vi "chooseOffensivePlay.vi"(8 "error in (no error)":errorcluster, 11 "Game":refnum<class "Game.lvclass">) -> (0 "error out":errorcluster, 2 "passFinishConditions":bool[](array[boolean]), 3 "Game out":refnum<class "Game.lvclass">, 4 "passdebug":T2[](array[typedef]), 5 "debugOffensivePlayFinished":T1[](array[typedef]))   [LabVIEW 2020, in "Game.lvclass"]
uses:
  Game.lvclass
  Team_class/OffensivePlay.ctl
  5RobotsPassGamePlay_class/PassFinishBallVelConditionDegub.ctl
  5RobotsPassGamePlay_class/PassFinishReceiverDistanceToBallConditionDebug.ctl
  Referee_class/command_interpreted.ctl
  Game.lvclass/Game.ctl
  Team_class/Team.lvclass/Team.ctl
  Referee_class/Referee.lvclass/Referee.ctl
  StopOffensivePlay_class/StopOffensivePlay.lvclass
  PreparePenaltyEnemyPlay_class/PreparePenaltyEnemyPlay.lvclass
  EnemyPossessionAtEnemyFieldPlay_class/EnemyPossessionAtEnemyFieldPlay.lvclass
  EnemyPossessionAtOurFieldPlay_class/EnemyPossessionAtOurFieldPlay.lvclass
  PreparePenaltyAllyPlay_class/PreparePenaltyAllyPlay.lvclass
  KickPenaltyAllyPlay_class/KickPenaltyAllyPlay.lvclass
  PrepareKickoffAllyPlay_class/PrepareKickoffAllyPlay.lvclass
  PrepareKickoffEnemyPlay_class/PrepareKickoffEnemyPlay.lvclass
  SimplePass_class/SimplePass.lvclass
  PreparePassPlay_class/PreparePassPlay.lvclass
  PrepareRollToPassPlay_class/PrepareRollToPassPlay.lvclass
  PrepareDoublePassPlay_class/PrepareDoublePassPlay.lvclass
  PrepareTriplePassPlay_class/PrepareTriplePassPlay.lvclass
  PassToStriker_class/PassToStriker.lvclass
  PassTo2ndStriker_class/PassTo2ndStriker.lvclass
  KeeperPassToStrikerPlay_class/KeeperPassToStrikerPlay.lvclass
  TableWithStrikerPlay_class/TableWithStrikerPlay.lvclass
  TableWith2ndStrikerPlay_class/TableWith2ndStrikerPlay.lvclass
  ABCPassPlay_class/ABCPassPlay.lvclass
  ACBPassPlay_class/ACBPassPlay.lvclass
  DirectKickPlay_class/DirectKickPlay.lvclass
  DirectEnemyPlay_class/DirectEnemyPlay.lvclass
  NormalGamePlay_class/NormalGamePlay.lvclass
  PrepareKeeperPassPlay_class/PrepareKeeperPassPlay.lvclass
  PreparePassInGame1_class/PreparePassInGame1.lvclass
  5RobotsPassGamePlay_class/5RobotsPassGamePlay.lvclass
  5PreparePassGamePlay_class/5PreparePassGamePlay.lvclass
  5RobotsNormalGamePlay_class/5RobotsNormalGamePlay.lvclass
  5RobotsKeeperGame_class/5RobotsKeeperGame.lvclass
  TestPlay_class/TestPlay.lvclass
  BallOutOfFieldPlay_class/BallOutOfFieldPlay.lvclass
  Utilities_class/Utilities.lvclass
  Playbook_class/Playbook.lvclass/Playbook.ctl
  Playbook_class/Read offensive_plays.vi
  Playbook_class/Write offensive_plays.vi
  Read OffensiveTeam.vi
  Read Referee.vi
  Referee_class/Read command_interpreted.vi
  Team_class/Read OffensivePlay.vi
  Team_class/Write OffensivePlay.vi
  Write OffensiveTeam.vi
  Ally_class/Ally.lvclass
  Referee_class/Referee.lvclass
  Playbook_class/Playbook.lvclass
  Play_class/Play.lvclass
  IndirectEnemyPlay_class/IndirectEnemyPlay.lvclass
  PassPlay_class/PassPlay.lvclass
  HaltPlay_class/HaltPlay.lvclass
panel:
  in  "NewOffensivePlays":T3[](array[typedef])=[enum."TestPlay", enum."BallOutOfField", enum."StopOffensive", enum."Prepare Penalty Enemy", enum."PreparePenaltyAlly", enum."KickPenaltyAlly", enum."PrepareKickoffAlly", enum."PrepareKickoffEnemy", enum."DirectEnemy", enum."PreparePass", enum."EnemyPossesionAtOurField", enum."EnemyPossessionAtEnemyField", enum."5RobotsKeeperGame", enum."5RobotsPassGamePlay", enum."5PreparePassGame", enum."5RobotsNormalGamePlay"]
  in  "OldOffensivePlays":T3[](array[typedef])=[enum."TestPlay", enum."BallOutOfField", enum."StopOffensive", enum."Prepare Penalty Enemy", enum."PreparePenaltyAlly", enum."KickPenaltyAlly", enum."PrepareKickoffAlly", enum."PrepareKickoffEnemy", enum."DirectEnemy", enum."SimplePass", enum."PreparePass", enum."PrepareRollToPass", enum."PrepareDoublePass", enum."PassToStriker", enum."PassTo2ndStriker", enum."TableWithStriker", enum."TableWith2ndStrikerPlay", enum."DirectKick", enum."EnemyPossesionAtOurField", enum."EnemyPossessionAtEnemyField", enum."PrepareTriplePass", enum."ABCPass", enum."PrepareKeeperPass", enum."KeeperPassToStriker", enum."ACBPass", enum."NormalGame", enum."PreparePassInGame1", enum."5RobotsKeeperGame", enum."5RobotsPassGamePlay", enum."5RobotsNormalGamePlay"]
  in  "Game in":refnum<class "Game.lvclass">
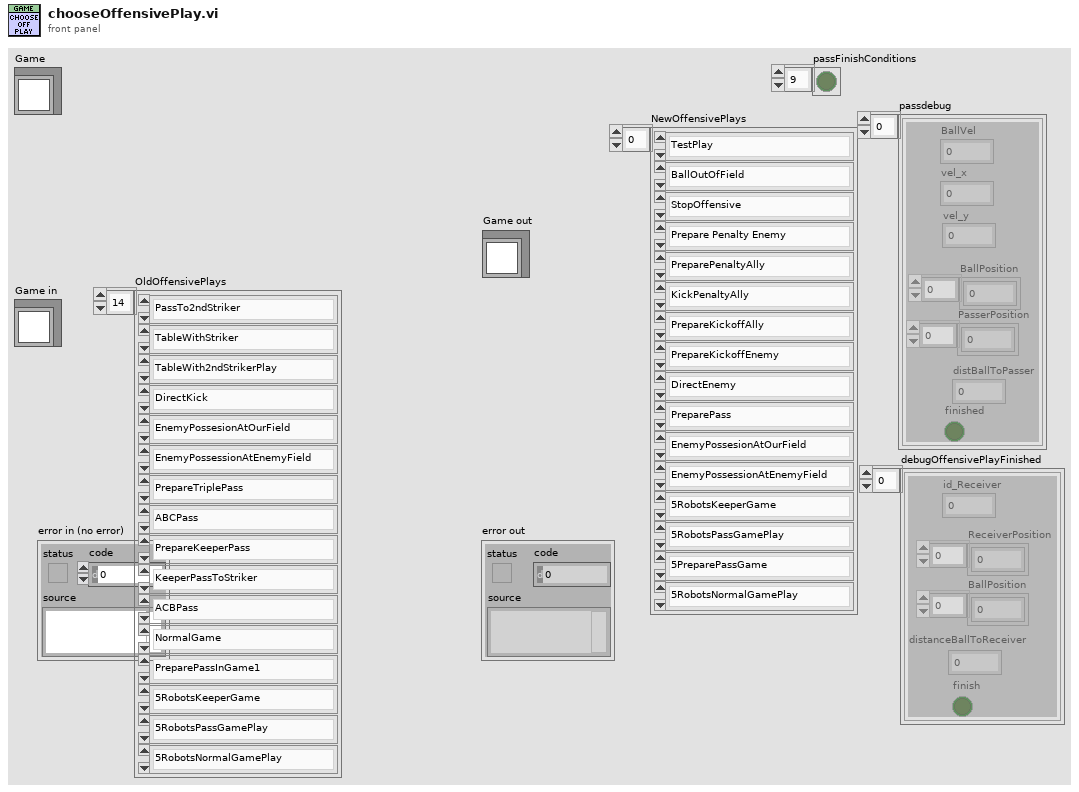
[diagram p1: front panel]
types:
  T1 = typedef "PassFinishReceiverDistanceToBallConditionDebug.ctl" = cluster{"id_Receiver":i32, "ReceiverPosition":dbl[], "BallPosition":dbl[], "distanceBallToReceiver":dbl, "finish":bool}
  T2 = typedef "PassFinishBallVelConditionDegub.ctl" = cluster{"BallVel":dbl, "BallPosition":dbl[], "PasserPosition":dbl[], "distBallToPasser":dbl, "finished":bool, "vel_x":dbl, "vel_y":dbl}
  T3 = typedef "OffensivePlay.ctl" = enum16{"5RobotsPassGamePlay", "5PreparePassGame", "5RobotsKeeperGame", "KeeperPassToStriker", "5RobotsNormalGamePlay", "PrepareKeeperPass", "ACBPass", "ABCPass", "PrepareTriplePass", "TableWithStriker", "TableWith2ndStrikerPlay", "PrepareDoublePass", "PrepareRollToPass", "SimplePass", "PreparePass", "PassToStriker", "BallOutOfField", "PassTo2ndStriker", "StopOffensive", "Prepare Penalty Enemy", "EnemyPossessionAtEnemyField", "EnemyPossesionAtOurField", "TestPlay", "PreparePenaltyAlly", "KickPenaltyAlly", "PrepareKickoffAlly", "PrepareKickoffEnemy", "IndirectEnemy", "DirectEnemy", "PreparePassInGame1", "NormalGame", "DirectKick", "Pass", "Halt", "Timeout", "PassPlay", "PenaltyEnemy"}
  T4 = typedef "command_interpreted.ctl" = enum16{"Goal Ally", "Goal Enemy", "Ball Placement Enemy", "Ball Placement Ally", "Normal Half Time", "Extra Time  Break", "Extra Half Time", "None", "Post Game", "PKA Normal Start", "Prepare Kickoff Ally", "PKE Normal Start", "Prepare Kickoff Enemy", "Force Start", "Halt", "Timeout", "Prepare Penalty Ally", "Prepare Penalty Enemy", "PPA NormalStart", "PPE Normal Start", "Indirect Free Ally", "Direct Free Enemy", "Direct Free Ally", "Indirect Free Enemy", "Stop"}
  T5 = typedef "offensive_plays.ctl" = cluster{"Play":refnum<class "Play.lvclass">, "TestPlay":refnum<class "TestPlay.lvclass">, "EnemyPossessionAtEnemyFieldPlay":refnum<class "EnemyPossessionAtEnemyFieldPlay.lvclass">, "EnemyPossessionAtOurFieldPlay":refnum<class "EnemyPossessionAtOurFieldPlay.lvclass">, "NormalGamePlay":refnum<class "NormalGamePlay.lvclass">, "IndirectEnemyPlay":refnum<class "IndirectEnemyPlay.lvclass">, "PrepareKickoffAllyPlay":refnum<class "PrepareKickoffAllyPlay.lvclass">, "PrepareKickoffEnemyPlay":refnum<class "PrepareKickoffEnemyPlay.lvclass">, "KickPenaltyAllyPlay":refnum<class "KickPenaltyAllyPlay.lvclass">, "PreparePenaltyAllyPlay":refnum<class "PreparePenaltyAllyPlay.lvclass">, "DirectEnemyPlay":refnum<class "DirectEnemyPlay.lvclass">, "PreparePenaltyEnemyPlay":refnum<class "PreparePenaltyEnemyPlay.lvclass">, "BallOutOfFieldPlay":refnum<class "BallOutOfFieldPlay.lvclass">, "StopOffensivePlay":refnum<class "StopOffensivePlay.lvclass">, "PassPlay":refnum<class "PassPlay.lvclass">, "DirectKickPlay":refnum<class "DirectKickPlay.lvclass">, "HaltPlay":refnum<class "HaltPlay.lvclass">, "PreparePassPlay":refnum<class "PreparePassPlay.lvclass">, "PassToStrikerPlay":refnum<class "PassToStriker.lvclass">, "PassTo2ndStrikerPlay":refnum<class "PassTo2ndStriker.lvclass">, "SimplePassPlay":refnum<class "SimplePass.lvclass">, "PrepareRollToPassPlay":refnum<class "PrepareRollToPassPlay.lvclass">, "PrepareDoublePassPlay":refnum<class "PrepareDoublePassPlay.lvclass">, "TableWith2ndStrikerPlay":refnum<class "TableWith2ndStrikerPlay.lvclass">, "TableWithStrikerPlay":refnum<class "TableWithStrikerPlay.lvclass">, "PrepareTriplePassPlay":refnum<class "PrepareTriplePassPlay.lvclass">, "ABCPassPlay":refnum<class "ABCPassPlay.lvclass">, "PreparePassInGame1":refnum<class "PreparePassInGame1.lvclass">, "ACBPassPlay":refnum<class "ACBPassPlay.lvclass">, "PrepareKeeperPassPlay":refnum<class "PrepareKeeperPassPlay.lvclass">, "KeeperPassToStrikerPlay":refnum<class "KeeperPassToStrikerPlay.lvclass">, "SimplePass":refnum<class "SimplePass.lvclass">, "SimplePass 2":refnum<class "SimplePass.lvclass">, "5RobotsNormalGamePlay":refnum<class "5RobotsNormalGamePlay.lvclass">, "5RobotsPassGamePlay":refnum<class "5RobotsPassGamePlay.lvclass">, "5RobotsKeeperGame":refnum<class "5RobotsKeeperGame.lvclass">, "5PreparePassGamePlay":refnum<class "5PreparePassGamePlay.lvclass">}
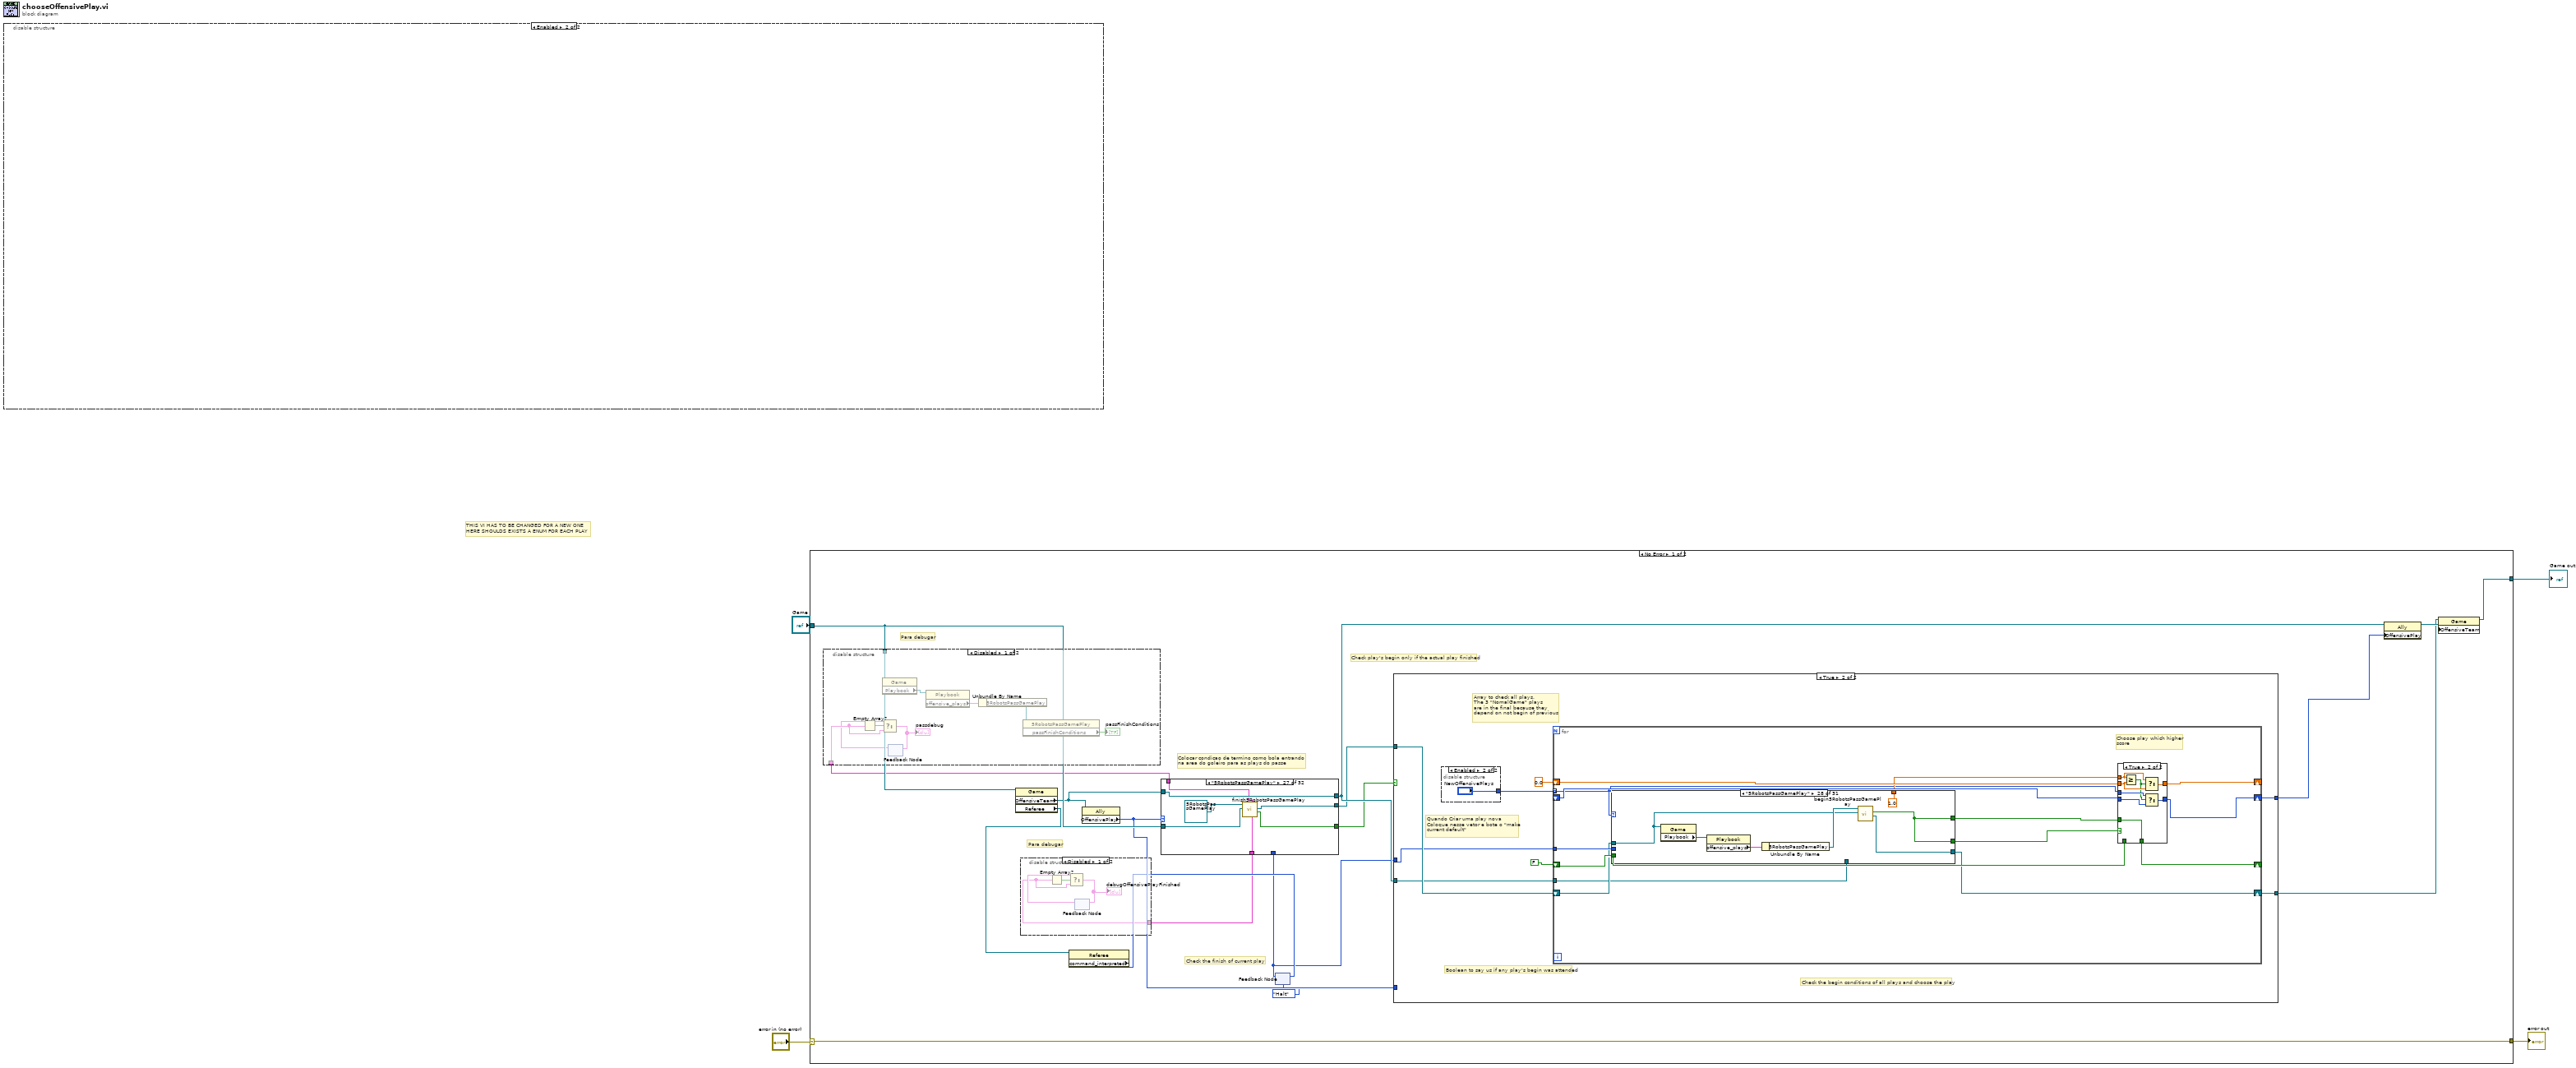
[diagram p0: block diagram]
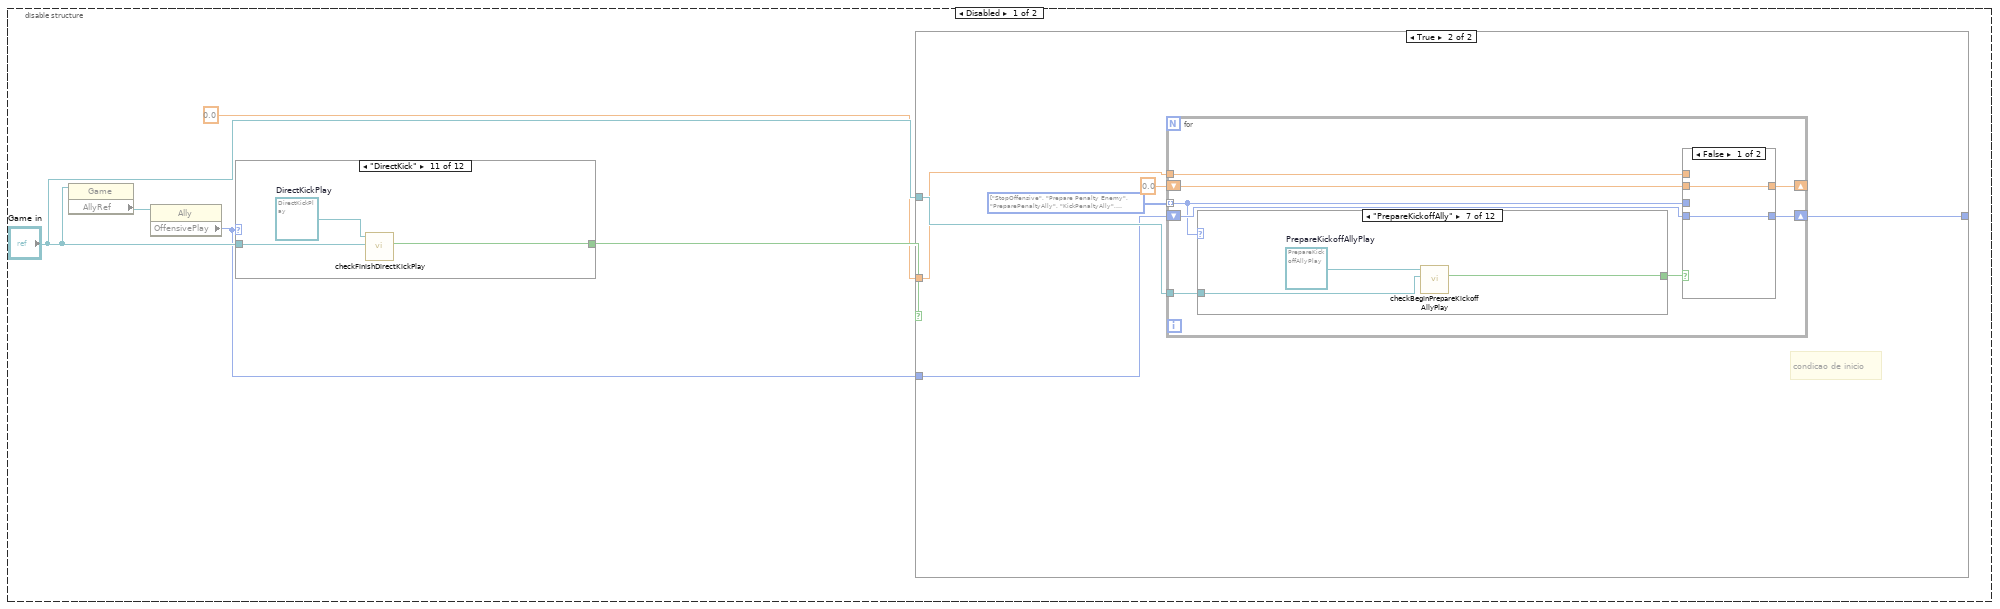
[diagram p2: hidden frame]
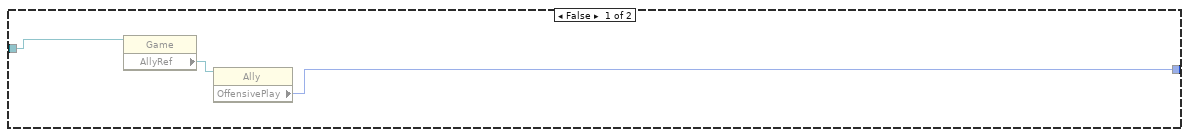
[diagram p3: hidden frame]
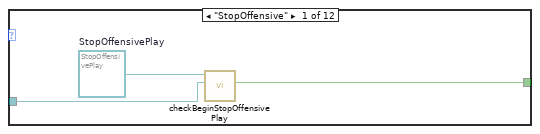
[diagram p4: hidden frame]
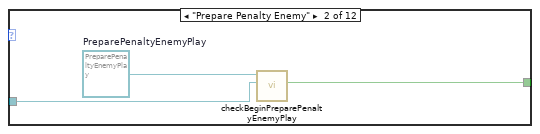
[diagram p5: hidden frame]
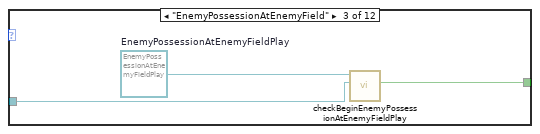
[diagram p6: hidden frame]
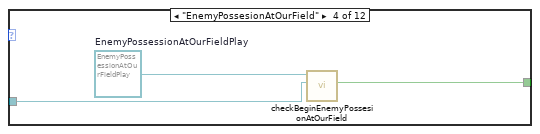
[diagram p7: hidden frame]
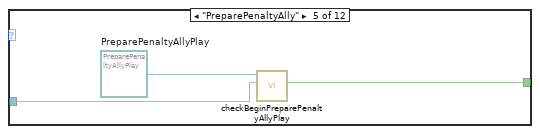
[diagram p8: hidden frame]
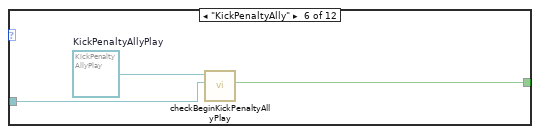
[diagram p9: hidden frame]
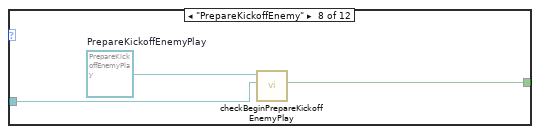
[diagram p10: hidden frame]
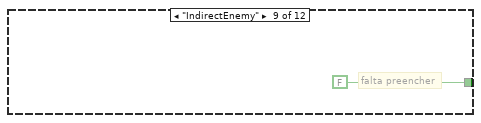
[diagram p11: hidden frame]
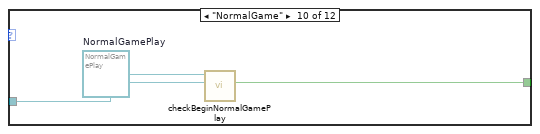
[diagram p12: hidden frame]
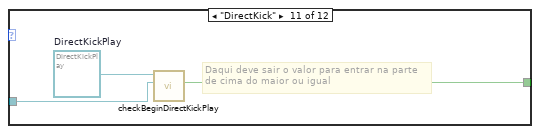
[diagram p13: hidden frame]
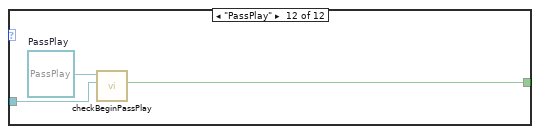
[diagram p14: hidden frame]
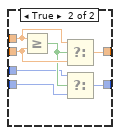
[diagram p15: hidden frame]
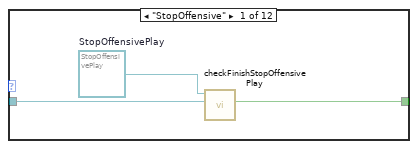
[diagram p16: hidden frame]
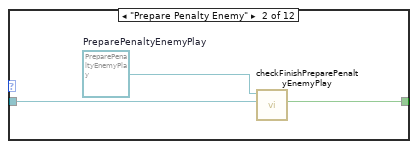
[diagram p17: hidden frame]
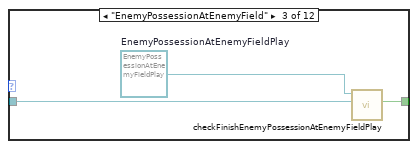
[diagram p18: hidden frame]
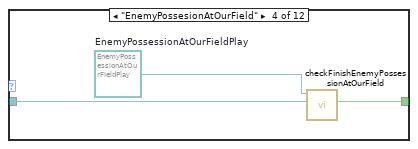
[diagram p19: hidden frame]
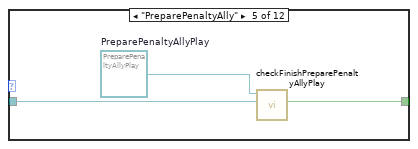
[diagram p20: hidden frame]
diagram:
  # "THIS VI HAS TO BE CHANGED FOR A NEW ONE\nHERE SHOULDS EXISTS A ENUM FOR EACH PLAY"
  n1 = disable-structure shown="Enabled" {
    frame Disabled {
      n2 = property class="Game"(reference="Game in") -> ("AllyRef"=w7:refnum<class "Ally.lvclass">)  [unwired: 1 in, 2 out]
      n3 = property class="Ally"(reference=w7) -> ("OffensivePlay"=w6:T3)  [unwired: 1 in, 2 out]
      n4 = case shown="\"DirectKick\"" w6 {
        tunnel: [w72 w74 w77 w80 w83 w86 w89 w92 FALSE w96 w99 w102] -> w9
        tunnel: "Game in" -> [w70 w75 w78 w81 w84 w87 w90 w93 _ w97 w100 w103]
        frame "StopOffensive" {
          w71 = refnum<class "StopOffensivePlay.lvclass"> refnum  # StopOffensivePlay
          n5 = call "checkFinishStopOffensivePlay.vi"("Game"=w70, "StopOffensivePlay in"=w71) -> ("Boolean"=w72:bool)  [unwired: 7 in, 2 out]
        }
        frame "Prepare Penalty Enemy" {
          w73 = refnum<class "PreparePenaltyEnemyPlay.lvclass"> refnum  # PreparePenaltyEnemyPlay
          n6 = call "checkFinishPreparePenaltyEnemyPlay.vi"("Game"=w75, "PreparePenaltyEnemyPlay in"=w73) -> ("Boolean"=w74:bool)  [unwired: 7 in, 2 out]
        }
        frame "EnemyPossessionAtEnemyField" {
          w76 = refnum<class "EnemyPossessionAtEnemyFieldPlay.lvclass"> refnum  # EnemyPossessionAtEnemyFieldPlay
          n7 = call "checkFinishEnemyPossessionAtEnemyFieldPlay.vi"("Game"=w78, "EnemyPossessionAtEnemyFieldPlay in"=w76) -> ("Boolean"=w77:bool)  [unwired: 7 in, 2 out]
        }
        frame "EnemyPossesionAtOurField" {
          w79 = refnum<class "EnemyPossessionAtOurFieldPlay.lvclass"> refnum  # EnemyPossessionAtOurFieldPlay
          n8 = call "checkFinishEnemyPossessionAtOurField.vi"("Game"=w81, "EnemyPossessionAtOurFieldPlay in"=w79) -> ("Boolean"=w80:bool)  [unwired: 7 in, 2 out]
        }
        frame "PreparePenaltyAlly" {
          w82 = refnum<class "PreparePenaltyAllyPlay.lvclass"> refnum  # PreparePenaltyAllyPlay
          n9 = call "checkFinishPreparePenaltyAllyPlay.vi"("Game"=w84, "PreparePenaltyAllyPlay in"=w82) -> ("Boolean"=w83:bool)  [unwired: 7 in, 2 out]
        }
        frame "KickPenaltyAlly" {
          w85 = refnum<class "KickPenaltyAllyPlay.lvclass"> refnum  # KickPenaltyAllyPlay
          n10 = call "checkFinishKickPenaltyAllyPlay.vi"("Game"=w87, "KickPenaltyAllyPlay in"=w85) -> ("Boolean"=w86:bool)  [unwired: 7 in, 2 out]
        }
        frame "PrepareKickoffAlly" {
          w88 = refnum<class "PrepareKickoffAllyPlay.lvclass"> refnum  # PrepareKickoffAllyPlay
          n11 = call "checkFinishPrepareKickoffAllyPlay.vi"("Game"=w90, "PrepareKickoffAllyPlay in"=w88) -> ("Boolean"=w89:bool)  [unwired: 7 in, 2 out]
        }
        frame "PrepareKickoffEnemy" {
          w91 = refnum<class "PrepareKickoffEnemyPlay.lvclass"> refnum  # PrepareKickoffEnemyPlay
          n12 = call "checkFinishPrepareKickoffEnemyPlay.vi"("Game"=w93, "PrepareKickoffEnemyPlay in"=w91) -> ("Boolean"=w92:bool)  [unwired: 7 in, 2 out]
        }
        frame "IndirectEnemy" {
          # "falta preencher"
        }
        frame "NormalGame" {
          w95 = refnum<class "NormalGamePlay.lvclass"> refnum  # NormalGamePlay
          n13 = call "checkFinishNormalGamePlay.vi"("Game"=w97, "NormalGamePlay in"=w95) -> ("finish?"=w96:bool)  [unwired: 6 in, 3 out]
        }
        frame "DirectKick" {
          w98 = refnum<class "DirectKickPlay.lvclass"> refnum  # DirectKickPlay
          n14 = call "checkFinishDirectKickPlay.vi"("Game"=w100, "DirectKickPlay in"=w98) -> ("Boolean"=w99:bool)  [unwired: 7 in, 2 out]
        }
        frame "PassPlay" {
          w101 = refnum<class "PassPlay.lvclass"> refnum  # PassPlay
          n15 = call "checkFinishPassPlay.vi"("Game"=w103, "PassPlay in"=w101) -> ("Boolean"=w102:bool)  [unwired: 7 in, 2 out]
        }
      }
      n16 = case shown="True" w9 {
        tunnel: "Game in" -> [w12 w17]
        tunnel: w6 -> [_ w16]
        tunnel: 0.0 -> [_ w14]
        tunnel: [w10 w13] -> _
        frame False {
          n17 = property class="Game"(reference=w12) -> ("AllyRef"=w11:refnum<class "Ally.lvclass">)  [unwired: 1 in, 2 out]
          n18 = property class="Ally"(reference=w11) -> ("OffensivePlay"=w10:T3)  [unwired: 1 in, 2 out]
        }
        frame True {
          w18 = T3[] [enum."StopOffensive", enum."Prepare Penalty Enemy", enum."PreparePenaltyAlly", enum."KickPenaltyAlly", enum."PrepareKickoffAlly", enum."PrepareKickoffEnemy", enum."IndirectEnemy", enum."DirectKick", enum."PassPlay", enum."EnemyPossessionAtEnemyField", enum."EnemyPossesionAtOurField", enum."NormalGame"] items=["5RobotsPassGamePlay", "5PreparePassGame", "5RobotsKeeperGame", "KeeperPassToStriker", "5RobotsNormalGamePlay", "PrepareKeeperPass", "ACBPass", "ABCPass", "PrepareTriplePass", "TableWithStriker", "TableWith2ndStrikerPlay", "PrepareDoublePass", "PrepareRollToPass", "SimplePass", "PreparePass", "PassToStriker", "BallOutOfField", "PassTo2ndStriker", "StopOffensive", "Prepare Penalty Enemy", "EnemyPossessionAtEnemyField", "EnemyPossesionAtOurField", "TestPlay", "PreparePenaltyAlly", "KickPenaltyAlly", "PrepareKickoffAlly", "PrepareKickoffEnemy", "IndirectEnemy", "DirectEnemy", "PreparePassInGame1", "NormalGame", "DirectKick", "Pass", "Halt", "Timeout", "PassPlay", "PenaltyEnemy"] ("appended array")
          # "condicao de inicio"
          n19 = for {
            tunnel: w18 -> [w22] mode=indexing
            shift-right: [w25] -> _
            shift-left: 0.0 -> [w24]
            tunnel: w17 -> [w21]
            shift-right: [w23] -> w13
            shift-left: w16 -> [w26]
            tunnel: w14 -> [w19]
            n20 = case shown="\"PrepareKickoffAlly\"" w22 {
              tunnel: w21 -> [w29 w32 w35 w38 w41 w44 w47 w50 _ w54 w57 w60]
              tunnel: [w28 w31 w34 w37 w40 w43 w46 w49 FALSE w53 w56 w59] -> w20
              frame "StopOffensive" {
                w27 = refnum<class "StopOffensivePlay.lvclass"> refnum  # StopOffensivePlay
                n21 = call "checkBeginStopOffensivePlay.vi"("Game"=w29, "StopOffensivePlay in"=w27) -> ("Boolean"=w28:bool)  [unwired: 7 in, 2 out]
              }
              frame "Prepare Penalty Enemy" {
                w30 = refnum<class "PreparePenaltyEnemyPlay.lvclass"> refnum  # PreparePenaltyEnemyPlay
                n22 = call "checkBeginPreparePenaltyEnemyPlay.vi"("Game"=w32, "PreparePenaltyEnemyPlay in"=w30) -> ("Boolean"=w31:bool)  [unwired: 7 in, 2 out]
              }
              frame "EnemyPossessionAtEnemyField" {
                w33 = refnum<class "EnemyPossessionAtEnemyFieldPlay.lvclass"> refnum  # EnemyPossessionAtEnemyFieldPlay
                n23 = call "checkBeginEnemyPossessionAtEnemyFieldPlay.vi"("Game"=w35, "EnemyPossessionAtEnemyFieldPlay in"=w33) -> ("Begin?"=w34:bool)  [unwired: 7 in, 2 out]
              }
              frame "EnemyPossesionAtOurField" {
                w36 = refnum<class "EnemyPossessionAtOurFieldPlay.lvclass"> refnum  # EnemyPossessionAtOurFieldPlay
                n24 = call "checkBeginEnemyPossesionAtOurField.vi"("Game"=w38, "EnemyPossessionAtOurFieldPlay in"=w36) -> ("Begin?"=w37:bool)  [unwired: 7 in, 2 out]
              }
              frame "PreparePenaltyAlly" {
                w39 = refnum<class "PreparePenaltyAllyPlay.lvclass"> refnum  # PreparePenaltyAllyPlay
                n25 = call "checkBeginPreparePenaltyAllyPlay.vi"("Game"=w41, "PreparePenaltyAllyPlay in"=w39) -> ("Boolean"=w40:bool)  [unwired: 7 in, 2 out]
              }
              frame "KickPenaltyAlly" {
                w42 = refnum<class "KickPenaltyAllyPlay.lvclass"> refnum  # KickPenaltyAllyPlay
                n26 = call "checkBeginKickPenaltyAllyPlay.vi"("Game"=w44, "KickPenaltyAllyPlay in"=w42) -> ("Boolean"=w43:bool)  [unwired: 7 in, 2 out]
              }
              frame "PrepareKickoffAlly" {
                w45 = refnum<class "PrepareKickoffAllyPlay.lvclass"> refnum  # PrepareKickoffAllyPlay
                n27 = call "checkBeginPrepareKickoffAllyPlay.vi"("Game"=w47, "PrepareKickoffAllyPlay in"=w45) -> ("Boolean"=w46:bool)  [unwired: 7 in, 2 out]
              }
              frame "PrepareKickoffEnemy" {
                w48 = refnum<class "PrepareKickoffEnemyPlay.lvclass"> refnum  # PrepareKickoffEnemyPlay
                n28 = call "checkBeginPrepareKickoffEnemyPlay.vi"("Game"=w50, "PrepareKickoffEnemyPlay in"=w48) -> ("Boolean"=w49:bool)  [unwired: 7 in, 2 out]
              }
              frame "IndirectEnemy" {
                # "falta preencher"
              }
              frame "NormalGame" {
                w52 = refnum<class "NormalGamePlay.lvclass"> refnum  # NormalGamePlay
                n29 = call "checkBeginNormalGamePlay.vi"(10:w54, "NormalGamePlay in"=w52) -> ("begin?"=w53:bool)  [unwired: 7 in, 2 out]
              }
              frame "DirectKick" {
                w55 = refnum<class "DirectKickPlay.lvclass"> refnum  # DirectKickPlay
                # "Daqui deve sair o valor para entrar na parte\nde cima do maior ou igual"
                n30 = call "checkBeginDirectKickPlay.vi"("Game"=w57, "DirectKickPlay in"=w55) -> ("Boolean"=w56:bool)  [unwired: 7 in, 2 out]
              }
              frame "PassPlay" {
                w58 = refnum<class "PassPlay.lvclass"> refnum  # PassPlay
                n31 = call "checkBeginPassPlay.vi"("Game"=w60, "PassPlay in"=w58) -> ("Boolean"=w59:bool)  [unwired: 7 in, 2 out]
              }
            }
            n32 = case shown="False" w20 {
              tunnel: w26 -> [w61 w63]
              tunnel: [w62 w69] -> w25
              tunnel: w24 -> [w62 w67]
              tunnel: w19 -> [_ w68]
              tunnel: w22 -> [_ w64]
              tunnel: [w61 w65] -> w23
              frame False {
              }
              frame True {
                n33 = Greater Or Equal?(x=w68, y=w67) -> (x >= y?=w66:bool)
                n34 = Select(t=w68, s=w66, f=w67) -> (s? t:f=w69:dbl)
                n35 = Select(t=w64, s=w66, f=w63) -> (s? t:f=w65:T3)
              }
            }
          }
        }
      }
    }
    frame Enabled {
    }
  }
  n36 = case shown="No Error" "error in (no error)" {
    selector: "error in (no error)" -> [w120 w506]
    tunnel: [w120 w506] -> w3
    tunnel: [w119 w505] -> w2
    tunnel: "Game" -> [w117 w505]
    frame No Error {
      # "Para debugar"
      # "Para debugar"
      # "Colocar condicao de termino como bola entrando\nna area do goleiro para as plays do passe"
      # "Check play's begin only if the actual play finished"
      # "Check the finish of current play"
      n37 = property class="Game"(reference=w117) -> ("OffensiveTeam"=w108:refnum<class "Ally.lvclass">, "Referee"=w112:refnum<class "Referee.lvclass">)  [unwired: 1 in, 2 out]
      n38 = property class="Referee"(reference=w112) -> ("command_interpreted"=w111:T4)  [unwired: 1 in, 2 out]
      n39 = property class="Ally"(reference=w108) -> ("OffensivePlay"=w113:T3)  [unwired: 1 in, 2 out]
      n40 = feedback #1(command_interpreted."Halt" ("command_interpreted")) -> (w109:T4)
      n41 = case shown="\"5RobotsPassGamePlay\"" w113 {
        tunnel: [w136 w141 w146 w151 w156 w160 w165 w170 w174 w178 w183 w188 w192 w196 w200 w203 w209 w213 w216 w220 w225 w229 w234 w239 w244 w251 w253 w260 w266 w272 w278 w282] -> w107
        tunnel: w117 -> [w134 w138 w142 w147 w152 w157 w161 w166 w171 w175 w180 w184 w189 w194 w198 w202 w207 w211 w215 w219 w223 w227 w231 w236 w242 w247 w257 w263 w265 w271 w276 w280]
        tunnel: w109 -> [_ _ w144 w149 w154 _ w163 w168 _ _ _ _ _ _ _ w204 _ _ _ _ _ _ w233 w240 w245 w250 _ w261 w268 w273 _ _]
        tunnel: w108 -> [w135 w139 w143 w148 w153 w158 w162 w167 w172 w177 w181 w185 w190 w195 w199 w205 w208 w212 w217 w221 w224 w228 w232 w238 w243 w248 w258 w262 w269 w275 w277 w281]
        tunnel: [w135 w139 w143 w148 w153 w158 w162 w167 w172 w176 w181 w186 w191 w195 w199 w205 w208 w212 w217 w221 w224 w228 w232 w237 w243 w249 w258 w262 w267 w275 w277 w281] -> w115
        tunnel: [w134 w138 w142 w147 w152 w157 w161 w166 w171 w175 w180 w184 w189 w194 w198 w202 w207 w211 w215 w219 w223 w227 w231 w236 w242 w247 w256 w263 w265 w271 w276 w280] -> w106
        tunnel: [_ _ _ _ _ _ _ _ _ _ _ _ _ _ _ _ _ _ _ _ _ _ _ _ _ _ w255 _ _ _ _ _] -> w105
        tunnel: [_ _ _ _ _ _ _ _ _ _ _ _ _ _ _ _ _ _ _ _ _ _ _ _ _ _ w254 _ _ _ _ _] -> w104
        frame "StopOffensive" {
          w137 = refnum<class "StopOffensivePlay.lvclass"> refnum  # StopOffensivePlay
          n42 = call "checkFinishStopOffensivePlay.vi"("Game"=w134, "StopOffensivePlay in"=w137) -> ("Boolean"=w136:bool)  [unwired: 7 in, 2 out]
        }
        frame "Prepare Penalty Enemy" {
          w140 = refnum<class "PreparePenaltyEnemyPlay.lvclass"> refnum  # PreparePenaltyEnemyPlay
          n43 = call "checkFinishPreparePenaltyEnemyPlay.vi"("Game"=w138, "PreparePenaltyEnemyPlay in"=w140) -> ("Boolean"=w141:bool)  [unwired: 7 in, 2 out]
        }
        frame "EnemyPossessionAtEnemyField" {
          w145 = refnum<class "EnemyPossessionAtEnemyFieldPlay.lvclass"> refnum  # EnemyPossessionAtEnemyFieldPlay
          n44 = call "checkFinishEnemyPossessionAtEnemyFieldPlay.vi"("last command_interpreted"=w144, "Game"=w142, "EnemyPossessionAtEnemyFieldPlay in"=w145) -> ("Boolean"=w146:bool)  [unwired: 6 in, 2 out]
        }
        frame "EnemyPossesionAtOurField" {
          w150 = refnum<class "EnemyPossessionAtOurFieldPlay.lvclass"> refnum  # EnemyPossessionAtOurFieldPlay
          n45 = call "checkFinishEnemyPossessionAtOurField.vi"("last command_interpreted"=w149, "Game"=w147, "EnemyPossessionAtOurFieldPlay in"=w150) -> ("Boolean"=w151:bool)  [unwired: 6 in, 2 out]
        }
        frame "PreparePenaltyAlly" {
          w155 = refnum<class "PreparePenaltyAllyPlay.lvclass"> refnum  # PreparePenaltyAllyPlay
          n46 = call "checkFinishPreparePenaltyAllyPlay.vi"("last command_interpreted"=w154, "Game"=w152, "PreparePenaltyAllyPlay in"=w155) -> ("Boolean"=w156:bool)  [unwired: 6 in, 2 out]
        }
        frame "KickPenaltyAlly" {
          w159 = refnum<class "KickPenaltyAllyPlay.lvclass"> refnum  # KickPenaltyAllyPlay
          n47 = call "checkFinishKickPenaltyAllyPlay.vi"("Game"=w157, "KickPenaltyAllyPlay in"=w159) -> ("Boolean"=w160:bool)  [unwired: 7 in, 2 out]
        }
        frame "PrepareKickoffAlly" {
          w164 = refnum<class "PrepareKickoffAllyPlay.lvclass"> refnum  # PrepareKickoffAllyPlay
          n48 = call "checkFinishPrepareKickoffAllyPlay.vi"("last command_interpreted"=w163, "Game"=w161, "PrepareKickoffAllyPlay in"=w164) -> ("Boolean"=w165:bool)  [unwired: 6 in, 2 out]
        }
        frame "PrepareKickoffEnemy" {
          w169 = refnum<class "PrepareKickoffEnemyPlay.lvclass"> refnum  # PrepareKickoffEnemyPlay
          n49 = call "checkFinishPrepareKickoffEnemyPlay.vi"("last command_interpreted"=w168, "Game"=w166, "PrepareKickoffEnemyPlay in"=w169) -> ("Boolean"=w170:bool)  [unwired: 6 in, 2 out]
        }
        frame "SimplePass" {
          w173 = refnum<class "SimplePass.lvclass"> refnum  # SimplePass in
          n50 = call "finishSimplePassPlay.vi"("Game in"=w171, "SimplePass in"=w173) -> ("finishSimplePass?"=w174:bool)  [unwired: 7 in, 2 out]
        }
        frame "PreparePass" {
          w179 = refnum<class "PreparePassPlay.lvclass"> refnum  # PreparePassPlay
          n51 = call "finishPreparePassPlay.vi"("OffensiveTeam in"=w177, "Game"=w175, "PreparePassPlay in"=w179) -> ("OffensiveTeam out"=w176:refnum<class "Ally.lvclass">, "FinishPreparePass?"=w178:bool)  [unwired: 5 in, 2 out]
        }
        frame "PrepareRollToPass" {
          w182 = refnum<class "PrepareRollToPassPlay.lvclass"> refnum  # PrepareRollToPassPlay in
          n52 = call "finishPrepareRollToPassPlay.vi"("Game"=w180, "PrepareRollToPassPlay in"=w182) -> ("FinishPrepareRollToPass?"=w183:bool)  [unwired: 7 in, 2 out]
        }
        frame "PrepareDoublePass" {
          w187 = refnum<class "PrepareDoublePassPlay.lvclass"> refnum  # PrepareDoublePassPlay
          n53 = call "finishPrepareDoublePassPlay.vi"("OffensiveTeam in"=w185, "Game"=w184, "PrepareDoublePassPlay in"=w187) -> ("OffensiveTeam out"=w186:refnum<class "Ally.lvclass">, "FinishPrepareDoublePass?"=w188:bool)  [unwired: 5 in, 2 out]
        }
        frame "PrepareTriplePass" {
          w193 = refnum<class "PrepareTriplePassPlay.lvclass"> refnum  # PrepareTriplePassPlay
          n54 = call "finishPrepareTriplePassPlay.vi"("Game"=w189, "OffensiveTeam in"=w190, "PrepareTriplePassPlay in"=w193) -> ("OffensiveTeam out"=w191:refnum<class "Ally.lvclass">, "finish?"=w192:bool)  [unwired: 5 in, 2 out]
        }
        frame "PassToStriker" {
          w197 = refnum<class "PassToStriker.lvclass"> refnum  # PassToStriker
          n55 = call "finishPassToStrikerPlay.vi"("Game"=w194, "PassToStriker in"=w197) -> ("finishPassToStriker?"=w196:bool)  [unwired: 7 in, 2 out]
        }
        frame "PassTo2ndStriker" {
          w201 = refnum<class "PassTo2ndStriker.lvclass"> refnum  # PassTo2ndStriker
          n56 = call "finishPassTo2ndStrikerPlay.vi"("Game"=w198, "PassTo2ndStriker in"=w201) -> ("finishPassTo2ndStriker?"=w200:bool)  [unwired: 7 in, 2 out]
        }
        frame "KeeperPassToStriker" {
          n57 = call "finishKeeperPassToStriker.vi"("command_interpreted"=w204, "Game"=w202, "OffesiveTeam"=w205, "KeeperPassToStrikerPlay in"=refnum<class "KeeperPassToStrikerPlay.lvclass"> refnum) -> ("finishKeeperPassToStriker"=w203:bool)  [unwired: 6 in, 1 out]
        }
        frame "TableWithStriker" {
          w210 = refnum<class "TableWithStrikerPlay.lvclass"> refnum  # TableWith2ndStrikerPlay
          n58 = call "finishTableWithStrikerPlay.vi"("Game"=w207, "TableWithStrikerPlay in"=w210) -> ("finishTableWith2ndStriker?"=w209:bool)  [unwired: 8 in, 1 out]
        }
        frame "TableWith2ndStrikerPlay" {
          w214 = refnum<class "TableWith2ndStrikerPlay.lvclass"> refnum  # TableWith2ndStrikerPlay
          n59 = call "finishTableWith2ndStrikerPlay.vi"("Game"=w211, "TableWith2ndStrikerPlay in"=w214) -> ("finishTableWith2ndStriker?"=w213:bool)  [unwired: 8 in, 1 out]
        }
        frame "ABCPass" {
          w218 = refnum<class "ABCPassPlay.lvclass"> refnum  # ABCPassPlay
          n60 = call "finishABCPassPlay.vi"("Game in"=w215, "ABCPassPlay in"=w218) -> ("Boolean"=w216:bool)  [unwired: 7 in, 2 out]
        }
        frame "ACBPass" {
          w222 = refnum<class "ACBPassPlay.lvclass"> refnum  # ACBPassPlay
          n61 = call "finishACBPassPlay.vi"("Game in"=w219, "ACBPassPlay in"=w222) -> ("finishACBPass"=w220:bool)  [unwired: 8 in, 1 out]
        }
        frame "IndirectEnemy" {
          w226 = refnum<class "TableWithStrikerPlay.lvclass"> refnum  # TableWith2ndStrikerPlay
          n62 = call "finishTableWithStrikerPlay.vi"("Game"=w223, "TableWithStrikerPlay in"=w226) -> ("finishTableWith2ndStriker?"=w225:bool)  [unwired: 8 in, 1 out]
        }
        frame "DirectKick" {
          w230 = refnum<class "DirectKickPlay.lvclass"> refnum  # DirectKickPlay
          n63 = call "finishDirectKickPlay.vi"("Game"=w227, "DirectKickPlay in"=w230) -> ("result"=w229:bool)  [unwired: 7 in, 2 out]
        }
        frame "DirectEnemy" {
          w235 = refnum<class "DirectEnemyPlay.lvclass"> refnum  # DirectEnemyPlay
          n64 = call "checkFinishDirectEnemyPlay.vi"("last command_interpreted"=w233, "Game"=w231, "DirectEnemyPlay in"=w235) -> ("Boolean"=w234:bool)  [unwired: 6 in, 2 out]
        }
        frame "NormalGame" {
          w241 = refnum<class "NormalGamePlay.lvclass"> refnum  # NormalGamePlay
          n65 = call "checkFinishNormalGamePlay.vi"("OffensiveTeam"=w238, "last command_interpreted"=w240, "Game"=w236, "NormalGamePlay in"=w241) -> ("OffensiveTeam out"=w237:refnum<class "Ally.lvclass">, "finish?"=w239:bool)  [unwired: 4 in, 2 out]
        }
        frame "PrepareKeeperPass" {
          n66 = call "finishPrepareKeeperPassPlay.vi"("Game"=w242, "command_interpreted"=w245, "PrepareKeeperPassPlay in"=refnum<class "PrepareKeeperPassPlay.lvclass"> refnum) -> ("finished ?"=w244:bool)  [unwired: 6 in, 2 out]
        }
        frame "PreparePassInGame1" {
          w252 = refnum<class "PreparePassInGame1.lvclass"> refnum  # PreparePassInGame1
          n67 = call "finishPreparePassInGame1.vi"("OffensiveTeam in"=w248, "command_interpreted"=w250, "Game in"=w247, "PreparePassInGame1 in"=w252) -> ("finished?"=w251:bool, "OffensiveTeam out"=w249:refnum<class "Ally.lvclass">)  [unwired: 4 in, 2 out]
        }
        frame "5RobotsPassGamePlay" {
          n68 = call-dynamic "finish5RobotsPassGamePlay.vi"("Game in"=w257, "5RobotsPassGamePlay in"=refnum<class "5RobotsPassGamePlay.lvclass"> refnum ("5RobotsPassGamePlay")) -> ("finish?"=w253:bool, "Game out"=w256:refnum<class "Game.lvclass">, "debugOffensivePlayFinished"=w254:T1[], "degugBallVel"=w255:T2[])  [unwired: 4 in, 2 out]
        }
        frame "5PreparePassGame" {
          n69 = call-dynamic "finish5PreparePassGamePlay.vi"("last_command"=w261, "Game"=w263, "5PreparePassGamePlay in"=refnum<class "5PreparePassGamePlay.lvclass"> refnum ("5PreparePassGamePlay")) -> ("result"=w260:bool)  [unwired: 6 in, 2 out]
        }
        frame "5RobotsNormalGamePlay", Default {
          n70 = call-dynamic "finish5RobotsNormalGamePlay.vi"("OffensiveTeam"=w269, "last command_interpreted"=w268, "Game"=w265, "5RobotsNormalGamePlay in"=refnum<class "5RobotsNormalGamePlay.lvclass"> refnum ("5RobotsNormalGamePlay")) -> ("OffensiveTeam out"=w267:refnum<class "Ally.lvclass">, "finish?"=w266:bool)  [unwired: 4 in, 2 out]
        }
        frame "5RobotsKeeperGame" {
          n71 = call-dynamic "finish5RobotsKeeperGame.vi"("Game"=w271, "command_interpreted"=w273, "5RobotsKeeperGame in"=refnum<class "5RobotsKeeperGame.lvclass"> refnum) -> ("finish?"=w272:bool)  [unwired: 6 in, 2 out]
        }
        frame "TestPlay" {
          w279 = refnum<class "TestPlay.lvclass"> refnum  # TestPlay
          n72 = call "checkFinishTestPlay.vi"("Game"=w276, "TestPlay in"=w279) -> ("Boolean"=w278:bool)  [unwired: 7 in, 2 out]
        }
        frame "BallOutOfField" {
          w283 = refnum<class "BallOutOfFieldPlay.lvclass"> refnum  # BallOutOfFieldPlay
          n73 = call "checkFinishBallOutOfFieldPlay.vi"("Game"=w280, "BallOutOfFieldPlay in"=w283) -> ("Finish Ball Out?"=w282:bool)  [unwired: 7 in, 2 out]
        }
      }
      n74 = disable-structure shown="Disabled" {
        disable-tunnel: w117 -> [w129 _]
        disable-tunnel: w105 -> [w123 _]
        frame Disabled {
          n75 = Empty Array?(array=w123) -> (empty?=w124:bool)
          n76 = property class="Game"(reference=w129) -> ("Playbook"=w128:refnum<class "Playbook.lvclass">)  [unwired: 1 in, 2 out]
          n77 = feedback #2() -> (w121:T2[])  [unwired: 1 in]
          n78 = Select(t=w121, s=w124, f=w123) -> (s? t:f=w122:T2[])
          "passdebug" <- w122
          n79 = feedback-in #2(w122) -> ()
          n80 = property class="Playbook"(reference=w128) -> ("offensive_plays"=w127:T5)  [unwired: 1 in, 2 out]
          n81 = Unbundle By Name(w127) -> ("5RobotsPassGamePlay"=w126:refnum<class "5RobotsPassGamePlay.lvclass">)
          n82 = property class="5RobotsPassGamePlay"(reference=w126) -> ("passFinishConditions"=→"passFinishConditions":bool[])  [unwired: 1 in, 2 out]
        }
        frame Enabled {
        }
      }
      n83 = disable-structure shown="Disabled" {
        disable-tunnel: w104 -> [w130 _]
        frame Disabled {
          n84 = Empty Array?(array=w130) -> (empty?=w133:bool)
          n85 = feedback #3() -> (w131:T1[])  [unwired: 1 in]
          n86 = Select(t=w131, s=w133, f=w130) -> (s? t:f=w132:T1[])
          "debugOffensivePlayFinished" <- w132
          n87 = feedback-in #3(w132) -> ()
        }
        frame Enabled {
        }
      }
      n88 = feedback-in #1(w111) -> ()
      n89 = case shown="True" w107 {
        tunnel: w113 -> [w285 _]
        tunnel: w106 -> [w284 w293]
        tunnel: [w285 w287] -> w114
        tunnel: w109 -> [_ w289]
        tunnel: w115 -> [_ w288]
        tunnel: [w284 w286] -> w116
        frame False {
        }
        frame True {
          # "Quando Criar uma play nova\nColoque nesse vetor e bote o \"make\ncurrent default\""
          # "Boolean to say us if any play's begin was attended"
          # "Array to check all plays.\nThe 3 \"NomalGame\" plays\nare in the final because they\ndepend on not begin of previous"
          # "Check the begin conditions of all plays and choose the play"
          n90 = disable-structure shown="Enabled" {
            disable-tunnel: ["OldOffensivePlays" "NewOffensivePlays"] -> w290
            frame Disabled {
            }
            frame Enabled {
            }
          }
          n91 = for {
            tunnel: w290 -> [w298] mode=indexing
            shift-right: [w308] -> _
            shift-left: 0.0 -> [w307]
            shift-right: [w297] -> w287
            shift-left: _ -> [w309]
            shift-right: [w305] -> _
            shift-left: FALSE -> [w303]
            tunnel: w289 -> [w302]
            tunnel: w288 -> [w296]
            shift-right: [w299] -> w286
            shift-left: w293 -> [w300]
            # "Choose play which higher\nscore"
            n92 = case shown="\"5RobotsPassGamePlay\"" w298 {
              selector: w298 -> [_ _ w323 _ w336 w343 w348 w354 _ w369 w374 w378 w383 _ _ _ _ _ _ _ _ _ _ _ _ w453 w461 _ _ _ _]
              tunnel: w300 -> [w310 w315 w320 w326 w332 w339 w345 w352 w359 w364 w370 w376 w382 w388 w392 w396 w401 w408 w415 w420 w424 w429 w436 w440 w444 w450 w459 w467 w474 w479 w490]
              tunnel: [w311 w314 w322 w327 w334 w341 w347 w353 w361 w365 w371 w380 w387 w389 w393 w397 w402 w409 w416 w421 w425 w430 w435 w439 w445 w452 w458 w465 w472 w478 w491] -> w304
              tunnel: [1.0 ("Score out") 2.0 w321 0.0 w333 w340 w346 w355 0.0 w366 w372 w379 w384 0.0 0.0 0.0 0.0 0.0 0.0 0.0 0.0 0.0 1.0 ("Score out") -1.0 ("Score out") 0.0 -1.0 ("Score out") w460 1.0 ("Score out") 3.0 ("Score out") 2.0 ("Score out") w492] -> w306
              tunnel: w303 -> [_ _ _ _ _ _ _ _ _ _ _ _ _ _ _ _ w403 w410 _ _ _ _ w438 _ _ w455 w463 _ _ _ _]
              tunnel: w302 -> [_ w316 w325 w328 w337 w344 _ _ w362 _ _ _ _ _ _ w398 _ _ w417 _ w426 w431 _ w442 w446 _ _ _ w473 w480 _]
              tunnel: [w311 w314 w322 w327 w334 w341 w347 w353 w361 w365 w371 w380 w387 w389 w393 w397 w402 w409 w416 w421 w425 w430 w435 w439 w445 w452 w458 w465 w472 w478 w491] -> w301
              tunnel: [w310 w315 w320 w326 w332 w339 w345 w352 w359 w364 w370 w376 w382 w388 w392 w396 w401 w408 w415 w420 w424 w429 w436 w440 w444 w450 w459 w466 w474 w485 w490] -> w299
              tunnel: w296 -> [_ _ w319 _ w331 w338 _ _ _ _ _ _ _ _ _ _ _ _ _ _ _ _ _ _ _ w449 w457 _ _ _ _]
              frame "BallOutOfField" {
                w313 = refnum<class "BallOutOfFieldPlay.lvclass"> refnum  # BallOutOfFieldPlay
                n93 = call "checkBeginBallOutOfFieldPlay.vi"("Game"=w310, "BallOutOfFieldPlay in"=w313) -> ("ball_out"=w311:bool)  [unwired: 7 in, 2 out]
              }
              frame "SimplePass" {
                w314 = FALSE
                w317 = refnum<class "SimplePass.lvclass"> refnum  # SimplePass in
                n94 = call "beginSimplePassPlay.vi"("last command_interpreted"=w316, "Game in"=w315, "SimplePass in"=w317) -> ()  [unwired: 6 in, 3 out]
              }
              frame "PreparePass" {
                w324 = refnum<class "PreparePassPlay.lvclass"> refnum  # PreparePassPlay
                n95 = call "beginPreparePassPlay.vi"("last command_interpreted"=w325, "Game"=w320, "PreparePassPlay in"=w324) -> ("BeginPreparePass?"=w322:bool)  [unwired: 6 in, 2 out]
                n96 = call "preparePassScore.vi"("OffensiveTeam"=w319, "OffensivePlay"=w323, "Play in"=w324) -> ("score"=w321:dbl)  [unwired: 6 in, 2 out]
              }
              frame "PrepareRollToPass" {
                w329 = refnum<class "PrepareRollToPassPlay.lvclass"> refnum  # PrepareRollToPassPlay in
                n97 = call "beginPrepareRollToPassPlay.vi"("last command_interpreted"=w328, "Game"=w326, "PrepareRollToPassPlay in"=w329) -> ("BeginPrepareRollToPass?"=w327:bool)  [unwired: 6 in, 2 out]
              }
              frame "PrepareDoublePass" {
                w335 = refnum<class "PrepareDoublePassPlay.lvclass"> refnum  # PrepareDoublePassPlay
                n98 = call "beginPrepareDoublePassPlay.vi"("last command_interpreted"=w337, "Game"=w332, "PrepareDoublePassPlay in"=w335) -> ("BeginPrepareDoublePass?"=w334:bool)  [unwired: 7 in, 1 out]
                n99 = call "preparePassScore.vi"("OffensiveTeam"=w331, "OffensivePlay"=w336, "Play in"=w335) -> ("score"=w333:dbl)  [unwired: 6 in, 2 out]
              }
              frame "PrepareTriplePass" {
                w342 = refnum<class "PrepareTriplePassPlay.lvclass"> refnum  # PrepareTriplePassPlay
                n100 = call "beginPrepareTriplePassPlay.vi"("Game"=w339, "last command_interpreted"=w344, "PrepareTriplePassPlay in"=w342) -> ("Boolean"=w341:bool)  [unwired: 6 in, 2 out]
                n101 = call "preparePassScore.vi"("OffensiveTeam"=w338, "OffensivePlay"=w343, "Play in"=w342) -> ("score"=w340:dbl)  [unwired: 6 in, 2 out]
              }
              frame "PassToStriker" {
                w351 = refnum<class "PassToStriker.lvclass"> refnum  # PassToStriker
                n102 = call "beginPassToStrikerPlay.vi"("Game"=w345, "PassToStriker in"=w351) -> ("BeginPassToStriker?"=w347:bool, "PassToStriker out"=w349:refnum<class "PassToStriker.lvclass">)  [unwired: 7 in, 1 out]
                n103 = call "ChoosePass.vi"("OffensivePlay"=w348, "Stk/2ndStk"=enum16{"Striker", "2ndStriker"}."Striker", "Game"=w345, "Play in"=w349) -> ("Factor Pass"=w346:dbl)  [unwired: 5 in, 2 out]
              }
              frame "PassTo2ndStriker" {
                w358 = refnum<class "PassTo2ndStriker.lvclass"> refnum  # PassTo2ndStriker
                n104 = call "beginPassTo2ndStrikerPlay.vi"("Game"=w352, "PassTo2ndStriker in"=w358) -> ("beginPassTo2ndStriker?"=w353:bool, "PassTo2ndStriker out"=w357:refnum<class "PassTo2ndStriker.lvclass">)  [unwired: 7 in, 1 out]
                n105 = call "ChoosePass.vi"("OffensivePlay"=w354, "Stk/2ndStk"=enum16{"Striker", "2ndStriker"}."2ndStriker", "Game"=w352, "Play in"=w357) -> ("Factor Pass"=w355:dbl)  [unwired: 5 in, 2 out]
              }
              frame "KeeperPassToStriker" {
                w360 = refnum<class "KeeperPassToStrikerPlay.lvclass"> refnum  # KeeperPassToStrikerPlay in
                n106 = call "beginKepperPassToStriker.vi"("command_interpreted"=w362, "Game"=w359, "KeeperPassToStrikerPlay in"=w360) -> ("beginKeeperPassToStriker"=w361:bool)  [unwired: 6 in, 2 out]
              }
              frame "TableWithStriker" {
                w367 = refnum<class "TableWithStrikerPlay.lvclass"> refnum  # TableWithStrikerPlay in
                n107 = call "beginTableWithStrikerPlay.vi"("Game"=w364, "TableWithStrikerPlay in"=w367) -> ("BeginTableWithStriker?"=w365:bool)  [unwired: 8 in, 1 out]
                n108 = call-dynamic "FactorPass.vi"("OffensivePlay"=w369, "Game"=w364, "Utilities in"=refnum<class "Utilities.lvclass"> refnum) -> ("Critério de marcação Normalizado"=w366:dbl)  [unwired: 6 in, 2 out]
              }
              frame "TableWith2ndStrikerPlay" {
                w375 = refnum<class "TableWith2ndStrikerPlay.lvclass"> refnum  # TableWith2ndStrikerPlay
                n109 = call "beginTableWith2ndStikerPlay.vi"("Game"=w370, "TableWith2ndStrikerPlay in"=w375) -> ("BeginTableWith2ndStriker?"=w371:bool)  [unwired: 7 in, 2 out]
                n110 = call-dynamic "FactorPass.vi"("OffensivePlay"=w374, "Game"=w370, "Utilities in"=refnum<class "Utilities.lvclass"> refnum) -> ("Critério de marcação Normalizado"=w372:dbl)  [unwired: 6 in, 2 out]
              }
              frame "ABCPass" {
                w381 = refnum<class "ABCPassPlay.lvclass"> refnum  # ABCPassPlay
                n111 = call "beginABCPassPlay.vi"("Game in"=w376, "ABCPassPlay in"=w381) -> ("result"=w380:bool)  [unwired: 7 in, 2 out]
                n112 = call-dynamic "FactorPass.vi"("OffensivePlay"=w378, "Game"=w376, "Utilities in"=refnum<class "Utilities.lvclass"> refnum) -> ("Critério de marcação Normalizado"=w379:dbl)  [unwired: 6 in, 2 out]
              }
              frame "ACBPass" {
                w386 = refnum<class "ACBPassPlay.lvclass"> refnum  # ACBPassPlay
                n113 = call "beginACBPassPlay.vi"("Game in"=w382, "ACBPassPlay in"=w386) -> ("beginACBPass"=w387:bool)  [unwired: 7 in, 2 out]
                n114 = call-dynamic "FactorPass.vi"("OffensivePlay"=w383, "Game"=w382, "Utilities in"=refnum<class "Utilities.lvclass"> refnum) -> ("Critério de marcação Normalizado"=w384:dbl)  [unwired: 6 in, 2 out]
              }
              frame "DirectKick" {
                w391 = refnum<class "DirectKickPlay.lvclass"> refnum  # DirectKickPlay
                n115 = call "beginDirectKickPlay.vi"("Game"=w388, "DirectKickPlay in"=w391) -> ("beginDirectKick?"=w389:bool)  [unwired: 7 in, 2 out]
              }
              frame "StopOffensive" {
                w395 = refnum<class "StopOffensivePlay.lvclass"> refnum  # StopOffensivePlay
                n116 = call "checkBeginStopOffensivePlay.vi"("Game"=w392, "StopOffensivePlay in"=w395) -> ("Boolean"=w393:bool)  [unwired: 7 in, 2 out]
              }
              frame "Prepare Penalty Enemy" {
                w400 = refnum<class "PreparePenaltyEnemyPlay.lvclass"> refnum  # PreparePenaltyEnemyPlay
                n117 = call "checkBeginPreparePenaltyEnemyPlay.vi"("last command_interpreted"=w398, "Game"=w396, "PreparePenaltyEnemyPlay in"=w400) -> ("Boolean"=w397:bool)  [unwired: 6 in, 2 out]
              }
              frame "EnemyPossessionAtEnemyField" {
                w402 = FALSE
                w407 = refnum<class "EnemyPossessionAtEnemyFieldPlay.lvclass"> refnum  # EnemyPossessionAtEnemyFieldPlay
                n118 = call "checkBeginEnemyPossessionAtEnemyFieldPlay.vi"("Game"=w401, "EnemyPossessionAtEnemyFieldPlay in"=w407) -> ("Begin?"=w405:bool)  [unwired: 7 in, 2 out]
                n119 = Not(x=w403) -> (.not. x?=w404:bool)
                n120 = And(x=w405, y=w404) -> ()  [unwired: 1 out]
              }
              frame "EnemyPossesionAtOurField" {
                w414 = refnum<class "EnemyPossessionAtOurFieldPlay.lvclass"> refnum  # EnemyPossessionAtOurFieldPlay
                n121 = call "checkBeginEnemyPossesionAtOurField.vi"("Game"=w408, "EnemyPossessionAtOurFieldPlay in"=w414) -> ("Begin?"=w412:bool)  [unwired: 7 in, 2 out]
                n122 = Not(x=w410) -> (.not. x?=w411:bool)
                n123 = And(x=w412, y=w411) -> (x .and. y?=w409:bool)
              }
              frame "PreparePenaltyAlly" {
                w419 = refnum<class "PreparePenaltyAllyPlay.lvclass"> refnum  # PreparePenaltyAllyPlay
                n124 = call "checkBeginPreparePenaltyAllyPlay.vi"("last command_interpreted"=w417, "Game"=w415, "PreparePenaltyAllyPlay in"=w419) -> ("Boolean"=w416:bool)  [unwired: 6 in, 2 out]
              }
              frame "KickPenaltyAlly" {
                w423 = refnum<class "KickPenaltyAllyPlay.lvclass"> refnum  # KickPenaltyAllyPlay
                n125 = call "checkBeginKickPenaltyAllyPlay.vi"("Game"=w420, "KickPenaltyAllyPlay in"=w423) -> ("Boolean"=w421:bool)  [unwired: 7 in, 2 out]
              }
              frame "PrepareKickoffAlly" {
                w428 = refnum<class "PrepareKickoffAllyPlay.lvclass"> refnum  # PrepareKickoffAllyPlay
                n126 = call "checkBeginPrepareKickoffAllyPlay.vi"("last command_interpreted"=w426, "Game"=w424, "PrepareKickoffAllyPlay in"=w428) -> ("Boolean"=w425:bool)  [unwired: 6 in, 2 out]
              }
              frame "PrepareKickoffEnemy" {
                w433 = refnum<class "PrepareKickoffEnemyPlay.lvclass"> refnum  # PrepareKickoffEnemyPlay
                n127 = call "checkBeginPrepareKickoffEnemyPlay.vi"("last command_interpreted"=w431, "Game"=w429, "PrepareKickoffEnemyPlay in"=w433) -> ("Boolean"=w430:bool)  [unwired: 6 in, 2 out]
              }
              frame "5RobotsNormalGamePlay", Default {
                n128 = call-dynamic "begin5RobotsNormalGamePlay.vi"("AnyPlayChosen?"=w438, "5RobotsNormalGamePlay in"=refnum<class "5RobotsNormalGamePlay.lvclass"> refnum ("5RobotsNormalGamePlay")) -> ("begin?"=w435:bool)  [unwired: 7 in, 2 out]
              }
              frame "PrepareKeeperPass" {
                w439 = FALSE
                n129 = call "beginPrepareKeeperPassPlay.vi"("command_interpreted"=w442, "Game in"=w440, "PrepareKeeperPassPlay in"=refnum<class "PrepareKeeperPassPlay.lvclass"> refnum) -> ()  [unwired: 6 in, 3 out]
              }
              frame "DirectEnemy" {
                w447 = refnum<class "DirectEnemyPlay.lvclass"> refnum  # DirectEnemyPlay
                n130 = call "checkBeginDirectEnemyPlay.vi"("last command_interpreted"=w446, "Game"=w444, "DirectEnemyPlay in"=w447) -> ("Boolean"=w445:bool)  [unwired: 6 in, 2 out]
              }
              frame "NormalGame" {
                w452 = FALSE ("Test")
                w456 = refnum<class "NormalGamePlay.lvclass"> refnum  # NormalGamePlay
                n131 = call "checkBeginNormalGamePlay.vi"("AnyPlayChosen?"=w455, "NormalGamePlay in"=w456) -> ("NormalGamePlay out"=w454:refnum<class "NormalGamePlay.lvclass">)  [unwired: 7 in, 2 out]
                n132 = call "preparePassInGameScore.vi"("OffensivePlay"=w453, "OffensiveTeam"=w449, "Play in"=w454) -> ()  [unwired: 6 in, 3 out]
              }
              frame "PreparePassInGame1" {
                w458 = FALSE
                w464 = refnum<class "PreparePassInGame1.lvclass"> refnum  # PreparePassInGame1
                n133 = call "beginPreparePassInGame1.vi"("AnyPlayChosen?"=w463, "PreparePassInGame1 in"=w464) -> ("PreparePassInGame1 out"=w462:refnum<class "PreparePassInGame1.lvclass">)  [unwired: 7 in, 2 out]
                n134 = call "preparePassInGameScore.vi"("OffensivePlay"=w461, "OffensiveTeam"=w457, "Play in"=w462) -> ("score"=w460:dbl)  [unwired: 6 in, 2 out]
              }
              frame "5RobotsPassGamePlay" {
                n135 = property class="Game"(reference=w467) -> ("Playbook"=w470:refnum<class "Playbook.lvclass">)  [unwired: 1 in, 2 out]
                n136 = property class="Playbook"(reference=w470) -> ("offensive_plays"=w469:T5)  [unwired: 1 in, 2 out]
                n137 = Unbundle By Name(w469) -> ("5RobotsPassGamePlay"=w468:refnum<class "5RobotsPassGamePlay.lvclass">)
                n138 = call "begin5RobotsPassGamePlay.vi"("Game in"=w467, "5RobotsPassGamePlay in"=w468) -> ("Game out"=w466:refnum<class "Game.lvclass">, "begin"=w465:bool)  [unwired: 6 in, 2 out]
              }
              frame "5PreparePassGame" {
                n139 = call-dynamic "begin5PreparePassGamePlay.vi"("last command_interpreted"=w473, "Game"=w474, "5PreparePassGamePlay in"=refnum<class "5PreparePassGamePlay.lvclass"> refnum ("5PreparePassGamePlay")) -> ("BeginPreparePass?"=w472:bool)  [unwired: 6 in, 2 out]
              }
              frame "5RobotsKeeperGame" {
                n140 = property class="Game"(reference=w479) -> (reference out=w486:refnum<class "Game.lvclass">, "Playbook"=w489:refnum<class "Playbook.lvclass">)  [unwired: 1 in, 1 out]
                n141 = property class="Playbook"(reference=w489) -> (reference out=w487:refnum<class "Playbook.lvclass">, "offensive_plays"=w484:T5)  [unwired: 1 in, 1 out]
                n142 = call-dynamic "begin5RobotsKeeperGame.vi"("Game in"=w479, "command_interpreted"=w480, "5RobotsKeeperGame in"=refnum<class "5RobotsKeeperGame.lvclass"> refnum) -> ("begin?"=w478:bool, "5RobotsKeeperGame out"=w477:refnum<class "5RobotsKeeperGame.lvclass">)  [unwired: 6 in, 1 out]
                n143 = Bundle By Name(cluster=w484, "5RobotsKeeperGame"=w477) -> (w483:T5)
                n144 = property class="Playbook"(reference=w487, "offensive_plays"=w483) -> (reference out=w488:refnum<class "Playbook.lvclass">)  [unwired: 1 in, 1 out]
                n145 = property class="Game"(reference=w486, "Playbook"=w488) -> (reference out=w485:refnum<class "Game.lvclass">)  [unwired: 1 in, 1 out]
              }
              frame "TestPlay" {
                w493 = refnum<class "TestPlay.lvclass"> refnum  # TestPlay
                n146 = call "checkBeginTestPlay.vi"("Game"=w490, "TestPlay in"=w493) -> ("Test"=w491:bool, "Score out"=w492:dbl)  [unwired: 6 in, 2 out]
              }
            }
            n147 = case shown="True" w304 {
              tunnel: w309 -> [w495 w499]
              tunnel: [w496 w504] -> w308
              tunnel: w307 -> [w496 w502]
              tunnel: w306 -> [_ w503]
              tunnel: w298 -> [_ w500]
              tunnel: [w495 w501] -> w297
              tunnel: [w494 w497] -> w305
              tunnel: w303 -> [w494 _]
              tunnel: w301 -> [_ w497]
              frame False {
              }
              frame True {
                n148 = Greater Or Equal?(x=w503, y=w502) -> (x >= y?=w498:bool)
                n149 = Select(t=w503, s=w498, f=w502) -> (s? t:f=w504:dbl)
                n150 = Select(t=w500, s=w498, f=w499) -> (s? t:f=w501:T3)
              }
            }
          }
        }
      }
      n151 = property class="Ally"(reference=w115, "OffensivePlay"=w114) -> (reference out=w118:refnum<class "Ally.lvclass">)  [unwired: 1 in, 1 out]
      n152 = property class="Game"(reference=w116, "OffensiveTeam"=w118) -> (reference out=w119:refnum<class "Game.lvclass">)  [unwired: 1 in, 1 out]
    }
    frame Error {
    }
  }
  "error out" <- w3
  "Game out" <- w2
